vi "ConvertTextBasedCodeToLabVIEW_CreateInterfaceList.vi"(11 "Classes":T1[](array[typedef])) -> (3 "InterfaceItems":T13[](array[typedef]))   [LabVIEW 2012]
uses:
  <resource>/Framework/Providers/Open_GDS/ClassProviders/Common/ConvertTextToLv_SubVIs/ConvertTextBasedCodeToLabVIEW_MissingType.ctl
  <resource>/Framework/Providers/Open_GDS/ClassProviders/Common/ConvertTextToLv_SubVIs/ConvertTextBasedCodeToLabVIEW_MissingTypeIconType.ctl
  <resource>/Framework/Providers/Open_GDS/ClassProviders/Common/String/GDSString_ClassDescriptionType.ctl
  <resource>/Framework/Providers/Open_GDS/ClassProviders/Common/String/GDSString_AccessScopeModifierType.ctl
  <resource>/Framework/Providers/Open_GDS/ClassProviders/Common/String/GDSString_ModifierType.ctl
  <resource>/Framework/Providers/Open_GDS/ClassProviders/Common/String/GDSString_MethodDescriptionType.ctl
  <resource>/Framework/Providers/Open_GDS/ClassProviders/Common/CommonVIs/CommonVIs_AttributeType.ctl
  <resource>/Framework/Providers/Open_GDS/ClassProviders/Common/CommonVIs/CommonVIs_AttributeDataType.ctl
  <resource>/Framework/Providers/Open_GDS/ClassProviders/Common/CommonVIs/CommonVIs_PropertyType.ctl
  <resource>/Framework/Providers/Open_GDS/ClassProviders/Common/String/GDSString_ClassParentType.ctl
  <resource>/Framework/Providers/Open_GDS/ClassProviders/Common/String/GDSString_ClassType.ctl
  <resource>/Framework/Providers/Open_GDS/ClassProviders/Common/String/GDSString_ClassOwnerType.ctl
  <resource>/Framework/Providers/Open_GDS/ClassProviders/Common/CommonVIs/CommonVIs_EnumType.ctl
  <resource>/Framework/Providers/Open_GDS/ClassProviders/Common/CommonVIs/CommonVIs_StructType.ctl
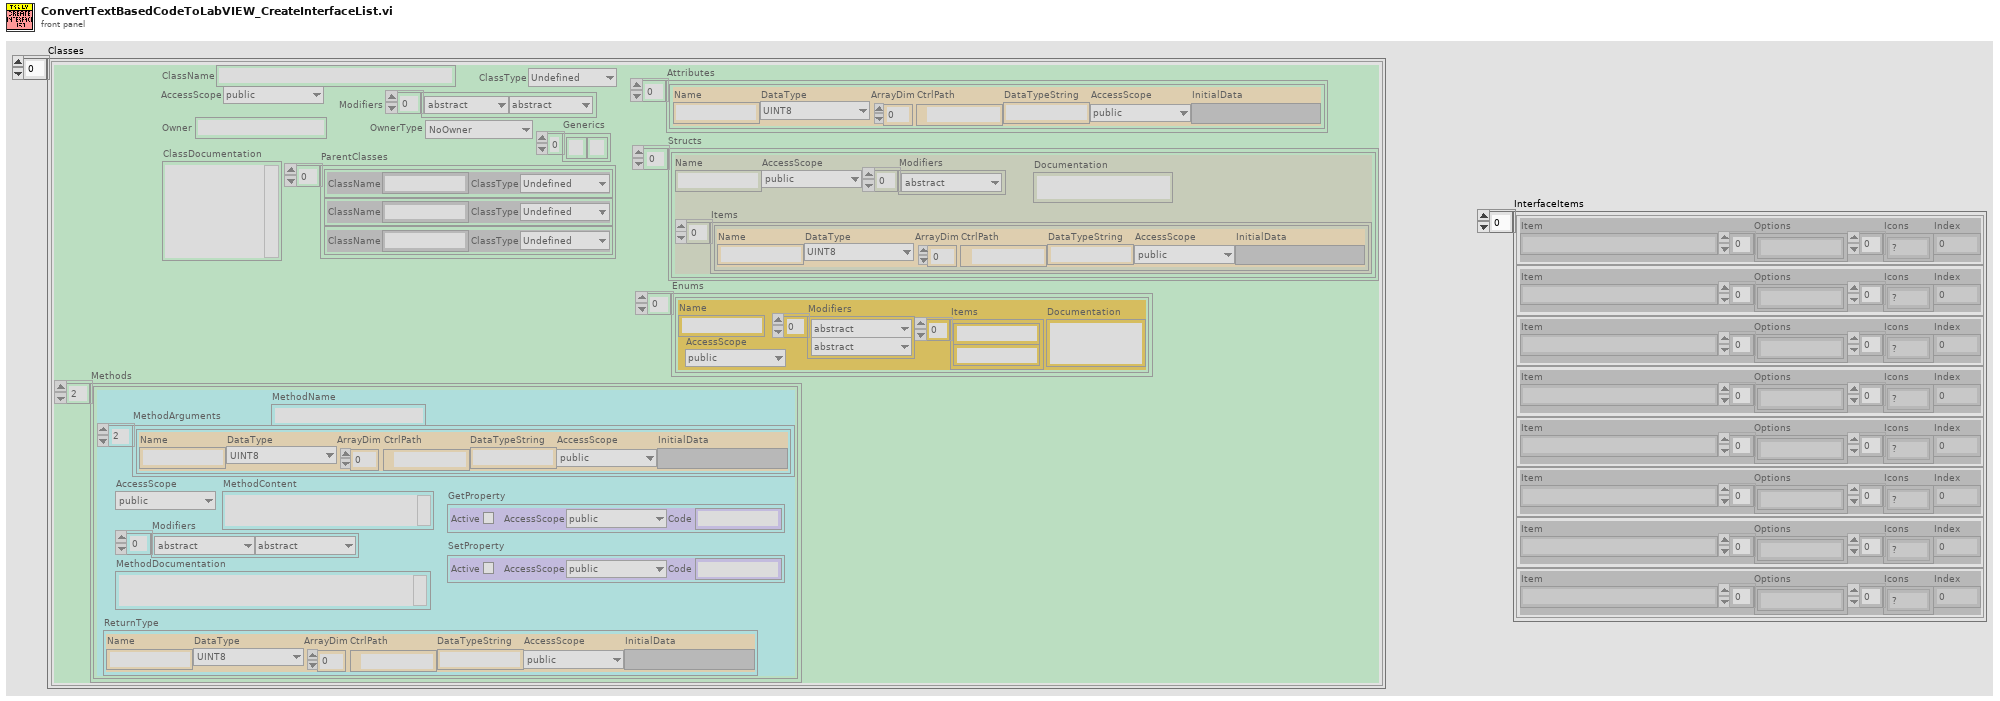
[diagram p1: front panel]
types:
  T1 = typedef "GDSString_ClassDescriptionType.ctl" = cluster{"ClassName":string, "AccessScope":T2, "Modifiers":T3[], "ClassDocumentation":string, "Methods":T4[], "ParentClasses":T8[], "ClassType":T9, "Owner":string, "OwnerType":T10, "Generics":string[], "Attributes":T5[], "Enums":T11[], "Structs":T12[]}
  T2 = typedef "GDSString_AccessScopeModifierType.ctl" = enum16{"public", "private", "protected", "internal"}
  T3 = typedef "GDSString_ModifierType.ctl" = enum16{"abstract", "static", "final", "synchronized", "strictfp", "async", "const", "event", "extern", "new", "native ", "override", "partial", "readonly", "sealed", "unsafe", "virtual", "volatile"}
  T4 = typedef "GDSString_MethodDescriptionType.ctl" = cluster{"ReturnType":T5, "MethodName":string, "AccessScope":T2, "Modifiers":T3[], "MethodDocumentation":string, "MethodContent":string, "MethodArguments":T5[], "GetProperty":T7, "SetProperty":T7}
  T5 = typedef "CommonVIs_AttributeType.ctl" = cluster{"Name":string, "DataType":T6, "ArrayDim":i32, "CtrlPath":path, "DataTypeString":string, "AccessScope":T2, "InitialData":variant}
  T6 = typedef "CommonVIs_AttributeDataType.ctl" = enum16{"UINT8", "INT8", "UINT16", "INT16", "UINT32", "INT32", "UINT64", "INT64", "SGL", "DBL", "EXT", "CSG", "CDB", "CXT", "TimeStamp", "STRING", "PATH", "BOOL", "ENUM", "RefNum", "VIRefNum", "LabVIEW Class", "Cluster", "Variant", "TypeDef", "Waveform", "LabVIEW Object", "Other", "void"}
  T7 = typedef "CommonVIs_PropertyType.ctl" = cluster{"Active":bool, "AccessScope":T2, "Code":string}
  T8 = typedef "GDSString_ClassParentType.ctl" = cluster{"ClassName":string, "ClassType":T9}
  T9 = typedef "GDSString_ClassType.ctl" = enum16{"Undefined", "Class", "Interface"}
  T10 = typedef "GDSString_ClassOwnerType.ctl" = enum16{"NoOwner", "Class", "Package/NameSpace"}
  T11 = typedef "CommonVIs_EnumType.ctl" = cluster{"Name":string, "AccessScope":T2, "Modifiers":T3[], "Items":string[], "Documentation":string}
  T12 = typedef "CommonVIs_StructType.ctl" = cluster{"Name":string, "AccessScope":T2, "Modifiers":T3[], "Items":T5[], "Documentation":string}
  T13 = typedef "ConvertTextBasedCodeToLabVIEW_MissingType.ctl" = cluster{"Item":string, "Options":string[], "Icons":T14[], "Index":i32}
  T14 = typedef "ConvertTextBasedCodeToLabVIEW_MissingTypeIconType.ctl" = enum16{"?", "Add", "Delete", "Implement", "Inherit"}
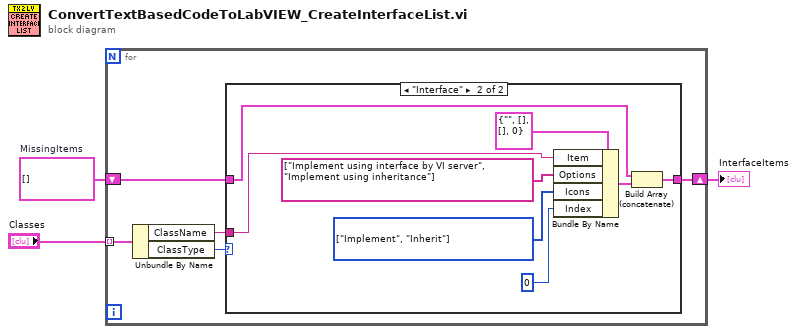
[diagram p0: block diagram]
diagram:
  w3 = T13[] []  # MissingItems
  n1 = for {
    shift-right: [w7] -> w2
    shift-left: w3 -> [w8]
    tunnel: "Classes" -> [w6] mode=indexing
    n2 = Unbundle By Name(w6) -> ("ClassName"=w4:string, "ClassType"=w5:T9)
    n3 = case shown="\"Interface\"" w5 {
      tunnel: w8 -> [w9 w17]
      tunnel: [w9 w16] -> w7
      tunnel: w4 -> [_ w10]
      frame Default {
      }
      frame "Interface" {
        w12 = T14[] [enum."Implement", enum."Inherit"] items=["?", "Add", "Delete", "Implement", "Inherit"] ("Icons")
        n4 = Bundle By Name(cluster=T13 {"Item"="", "Options"=[], "Icons"=[], "Index"=0} ("Cluster"), "Item"=w10, "Options"=string[] ["Implement using interface by VI server", "Implement using inheritance"], "Icons"=w12, "Index"=0 ("InitialIndex")) -> (w14:T13)
        n5 = Build Array (concatenate)(w17, w14) -> (w16:T13[])
      }
    }
  }
  "InterfaceItems" <- w2
